vi "CRYTime global.vi"() -> ()   [LabVIEW 2013]
panel:
  in  "Sweep type right":i32
  in  "Sweep type left":i32
  in  "Zero pad stimulus":cluster{"channel":i32, "true length":i32}
  in  "Attack right":sgl[](array[numeric]) format="%.2f"
  in  "Attack left":sgl[](array[numeric]) format="%.2f"
  in  "Discard cycles right":i32
  in  "Discard cycles left":i32
  in  "Sine waves right":cluster{"freq":dbl, "ampl":dbl, "cycles":dbl}[](array[cluster]) {"cycles" format="%.2f"; "ampl" format="%.2f"; "freq" format="%.2f"}
  in  "Sine waves left":cluster{"freq":dbl, "ampl":dbl, "cycles":dbl}[](array[cluster]) {"cycles" format="%.2f"; "ampl" format="%.2f"; "freq" format="%.2f"}
  in  "Output channel":i32
  in  "Cycles right":u32
  in  "Cycles left":u32
  in  "Level right":sgl format="%.2f"
  in  "Level left":sgl format="%.2f"
  in  "Response right":sgl[](array[numeric]) format="%.2f"
  in  "Response left":sgl[](array[numeric]) format="%.2f"
  in  "Stimulus right":sgl[](array[numeric]) format="%.2f"
  in  "Stimulus left":sgl[](array[numeric]) format="%.2f"
  # "not used anymore?"
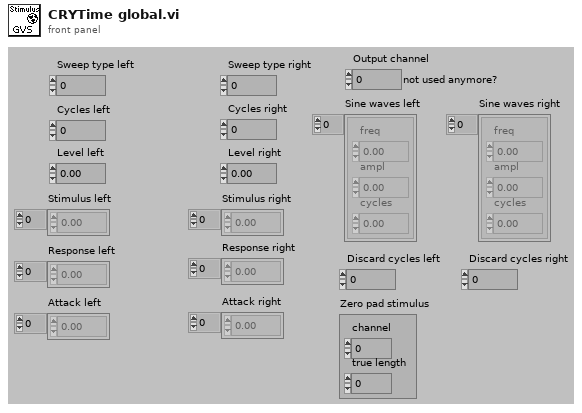
[diagram p1: front panel]
diagram:
